vi "温度检测系统.vi"() -> ()   [LabVIEW 2024]
uses:
  <vilib>/numeric/Random Number (Range) DBL.vi
  <vilib>/Utility/file.llb/Write Delimited Spreadsheet (DBL).vi
  <vilib>/ptbypt/NI_PtbyPt.lvlib
panel:
  out "越限次数":dbl
  in  "停止":bool
  out "状态显示":string
  out "最小值":dbl
  out "最大值":dbl
  out "均值":dbl
  out "采样点数":i32
  in  "通道切换":bool caption="A\n\nB"
  in  "温度下限":dbl
  in  "温度上限":dbl
  out "波形图表":cluster{"温度上限":dbl, "number":dbl, "温度下限":dbl}(graph)
  out "报警灯":bool
  out "当前温度":dbl(slide) caption="温度计" scale=0.0..100.0 scale format="%#.3g"
  # "仿真温度检测系统"
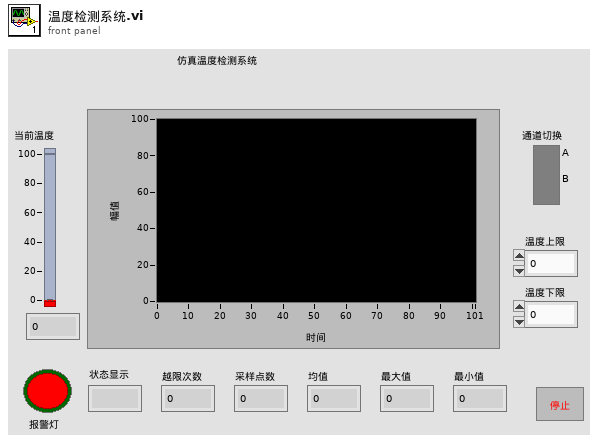
[diagram p1: front panel]
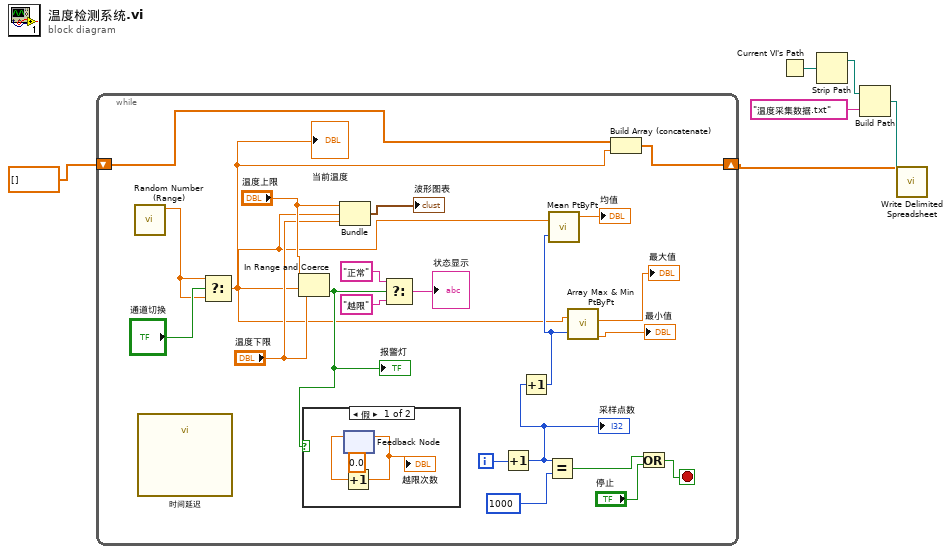
[diagram p0: block diagram]
diagram:
  n1 = while {
    shift-right: [w7] -> w1
    shift-left: dbl[] [] -> [w8]
    i -> [w28]
    stop <- w26 stop-if-true
    n2 = call-poly <vilib>:"Random Number (Range).vi"() -> ("number"=w13:dbl)  [unwired: 11 in]
    n3 = call "时间延迟"() -> ()  [unwired: 11 in, 1 out]
    n4 = Select(t=w13, s="通道切换", f=w13) -> (s? t:f=w9:dbl)
    "当前温度" <- w9
    n5 = In Range and Coerce(upper limit="温度上限", x=w9, lower limit="温度下限") -> (In Range?=w14:bool)  [unwired: 1 out]
    "报警灯" <- w14
    n6 = case shown="假" w14 {
      frame False {
        n7 = feedback #1(0.0) -> (w31:dbl)
        n8 = Increment(x=w31) -> (x+1=w29:dbl)
        "越限次数" <- w29
        n9 = feedback-in #1(w29) -> ()
      }
      frame True {
      }
    }
    n10 = Bundle("温度上限"="温度上限", "number"=w9, "温度下限"="温度下限") -> (→"波形图表":cluster{"温度上限":dbl, "number":dbl, "温度下限":dbl})  [unwired: 1 in]
    n11 = Select(t="正常", s=w14, f="越限") -> (s? t:f=→"状态显示":string)
    n12 = Increment(x=w28) -> (x+1=w16:i32)
    "采样点数" <- w16
    n13 = Increment(x=w16) -> (x+1=w15:i32)
    n14 = Equal?(x=w16, y=1000) -> (x = y?=w27:bool)
    n15 = call <vilib>:"Mean PtByPt.vi"("x"=w9, "sample length"=w15) -> ("mean"=→"均值":dbl)  [unwired: 2 in, 1 out]
    n16 = call <vilib>:"Array Max & Min PtByPt.vi"("input data point"=w9, "sample length"=w15) -> ("max value"=→"最大值":dbl, "min value"=→"最小值":dbl)  [unwired: 1 in, 3 out]
    n17 = Build Array (concatenate)(w8, w9) -> (w7:dbl[])
    n18 = Or(x=w27, y="停止") -> (x .or. y?=w26:bool)
  }
  n19 = Current VI's Path() -> (path=w3:path)
  n20 = Strip Path(path=w3) -> (stripped path=w5:path)  [unwired: 1 out]
  n21 = Build Path(base path=w5, name or relative path="温度采集数据.txt") -> (appended path=w6:path)
  n22 = call-poly <vilib>:"Write Delimited Spreadsheet.vi"("file path (dialog if empty)"=w6, "1D data"=w1) -> ()  [unwired: 12 in, 2 out]
